vi "Linear Interpolation Percent Open to GPM.vi"(10 "Percent":dbl) -> (2 "GPM":dbl)   [LabVIEW 2009]
uses:
  <vilib>/gmath/NI_Gmath.lvlib
panel:
  in  "Configuration":enum16{"DRK500,Station1", "DRK375,Lab"}(ring)
  # "Measured in test lab."
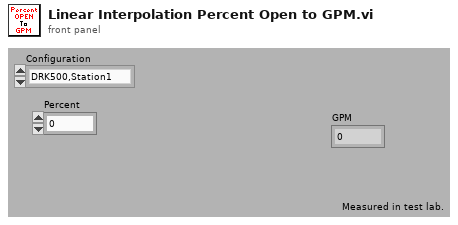
[diagram p1: front panel]
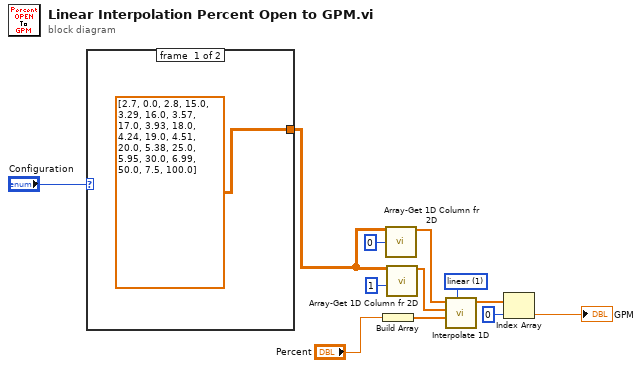
[diagram p0: block diagram]
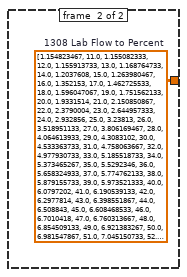
[diagram p2: hidden frame]
diagram:
  w12 = 1 items=["nearest", "linear", "spline", "cubic Hermite", "Lagrange"] ("method")
  n1 = case shown="\"DRK500,Station1\", Default" "Configuration" {
    tunnel: [dbl[][] [[2.7, 0.0], [2.8, 15.0], [3.29, 16.0], [3.57, 17.0], [3.93, 18.0], [4.24, 19.0], [4.51, 20.0], [5.38, 25.0], [5.95, 30.0], [6.99, 50.0], [7.5, 100.0]] ("DRK500 thru Small Flowmeter") w14] -> w1
    frame #0 {
    }
    frame #1 {
      w14 = dbl[][] [[1.154823467, 11.0], [1.155082333, 12.0], [1.155913733, 13.0], [1.168764733, 14.0], [1.2037608, 15.0], [1.263980467, 16.0], [1.352153, 17.0], [1.462725533, 18.0], [1.596047067, 19.0], [1.751562133, 20.0], [1.9331514, 21.0], [2.150850867, 22.0], [2.3790004, 23.0], [2.644957333, 24.0], [2.932856, 25.0], [3.23813, 26.0], [3.518951133, 27.0], [3.806169467, 28.0], [4.064613933, 29.0], [4.3083102, 30.0], [4.533363733, 31.0], [4.758063667, 32.0], [4.977930733, 33.0], [5.185518733, 34.0], [5.373465267, 35.0], [5.5292346, 36.0], [5.658324933, 37.0], [5.774762133, 38.0], [5.879155733, 39.0], [5.973521333, 40.0], [6.0797202, 41.0], [6.190539133, 42.0], [6.2977814, 43.0], [6.398551867, 44.0], [6.508843, 45.0], [6.608468533, 46.0], [6.7010418, 47.0], [6.760313667, 48.0], [6.854509133, 49.0], [6.921383267, 50.0], [6.981547867, 51.0], [7.045150733, 52.0], [7.1211556, 53.0], [7.153945267, 54.0], [7.1919082, 55.0], [7.221364733, 56.0], [7.2363738, 57.0], [7.2658748, 58.0], [7.290652133, 59.0], [7.306916267, 60.0], [7.328831, 61.0], [7.351323533, 62.0], [7.356630467, 63.0], [7.363471333, 64.0], [7.3759204, 65.0], [7.377457533, 66.0], [7.385319933, 67.0], [7.400870533, 68.0], [7.420039867, 69.0], [7.436503867, 70.0], [7.435100667, 71.0], [7.441507067, 72.0], [7.4586758, 73.0], [7.4709312, 74.0], [7.477849933, 75.0], [7.502882667, 76.0], [7.515599867, 77.0], [7.516479467, 78.0], [7.5161762, 79.0], [7.522149933, 80.0], [7.531457467, 81.0], [7.540166067, 82.0], [7.545417133, 83.0], [7.547076867, 84.0], [7.544551533, 85.0], [7.527355067, 86.0], [7.531499133, 87.0], [7.540953933, 88.0], [7.553015733, 89.0], [7.5680518, 90.0], [7.595900467, 91.0], [7.600769333, 92.0], [7.603110267, 93.0], [7.608227533, 94.0], [7.615357067, 95.0], [7.613050067, 96.0], [7.632628733, 97.0], [7.6430432, 98.0]]  # 1308 Lab Flow to Percent
    }
  }
  n2 = Build Array("Percent") -> (w9:dbl[])
  n3 = call "Array-Get 1D Column fr 2D.vi"("2D Array Data"=w1, "column index"=0) -> ("Column Data"=w4:dbl[])  [unwired: 13 in]
  n4 = call "Array-Get 1D Column fr 2D.vi"("2D Array Data"=w1, "column index"=1) -> ("Column Data"=w5:dbl[])  [unwired: 13 in]
  n5 = call <vilib>:"Interpolate 1D.vi"("method"=w12, "xi"=w9, "X"=w5, "Y"=w4) -> ("yi"=w8:dbl[])  [unwired: 5 in, 2 out]
  n6 = Index Array(array=w8, index=0) -> (element=→"GPM":dbl)
